vi "Lick.vi"(8 "error in (no error)":errorcluster, 10 "% decrease Thr":dbl[](array[numeric])=[10.0, 10.0, 10.0, 10.0, 10.0], 11 "Licker in":refnum<class "Licker.lvclass">) -> (0 "error out":errorcluster, 1 "Lick?":bool[](array[boolean]), 2 "data":waveform(dbl)[](array[waveform]), 3 "Licker out":refnum<class "Licker.lvclass">)   [LabVIEW 2014, in "Licker.lvclass"]
uses:
  Licker.lvclass
  Licker.lvclass/Licker.ctl
  <vilib>/Analysis/5stat.llb/RMS (DBL).vi
  <vilib>/DAQmx/read.llb/DAQmx Read.vi
  <vilib>/DAQmx/read.llb/DAQmx Read (Analog 1D Wfm NChan NSamp).vi
  <vilib>/Analysis/NI_AALPro.lvlib
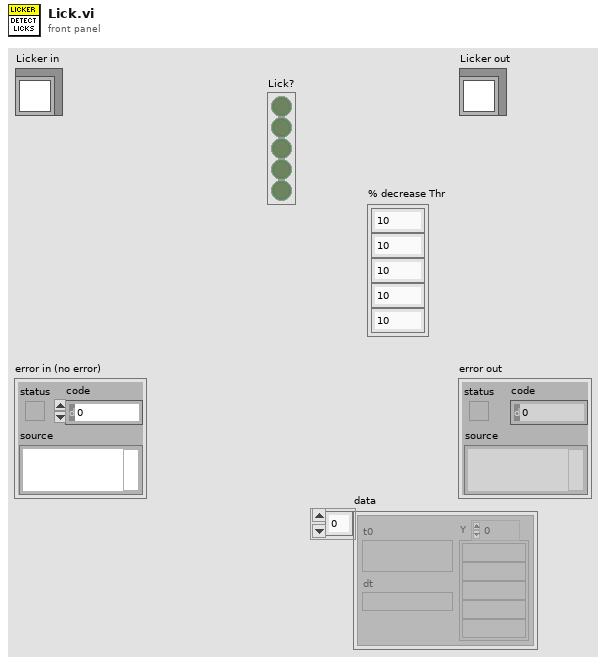
[diagram p1: front panel]
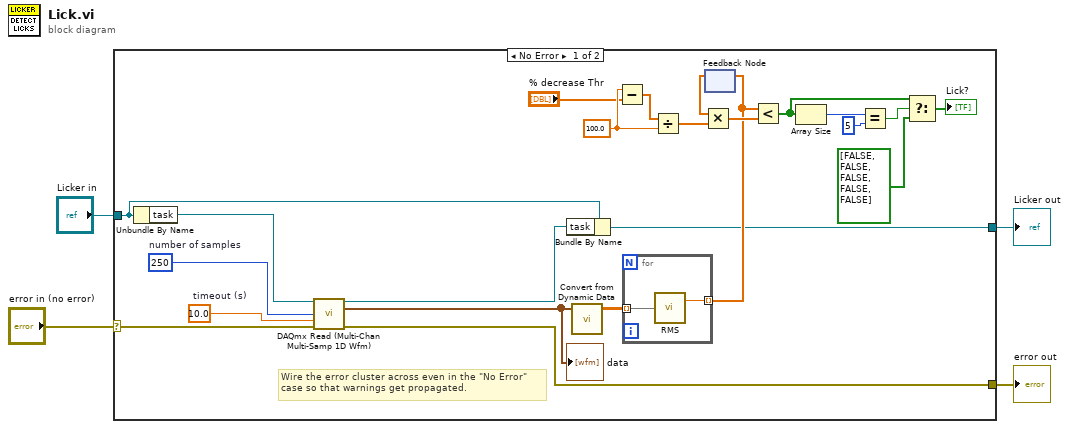
[diagram p0: block diagram]
diagram:
  n1 = case shown="No Error" "error in (no error)" {
    selector: "error in (no error)" -> [w17 w31]
    tunnel: [w16 w31] -> w3
    tunnel: [w13 w30] -> w1
    tunnel: "Licker in" -> [w14 w30]
    frame No Error {
      w18 = 250  # number of samples
      w21 = 100.0 ("y")
      w27 = 10.0  # timeout (s)
      # "Wire the error cluster across even in the \"No Error\"\ncase so that warnings get propagated."
      n2 = Unbundle By Name(w14) -> ("task"=w15:refnum<k21>)
      n3 = call-poly "DAQmx Read (Multi-Chan Multi-Samp 1D Wfm).vi"("task/channels in"=w15, "number of samples per channel"=w18, "timeout"=w27, "error in"=w17) -> ("task out"=w12:refnum<k21>, "data"=w26:waveform(dbl)[], "error out"=w16:errorcluster)  [unwired: 9 in]
      "data" <- w26
      n4 = Bundle By Name(cluster=w14, "task"=w12) -> (w13:refnum<class "Licker.lvclass">)
      n5 = call "Convert from Dynamic Data"("Dynamic Data Type"=w26) -> ("Array"=w25:dbl[][])  [unwired: 3 in]
      n6 = Subtract(x=w21, y="% decrease Thr") -> (x-y=w20:dbl[])
      n7 = for {
        tunnel: w25 -> [w29] mode=indexing
        tunnel: [w28] -> w19 mode=indexing
        n8 = call-poly <vilib>:"RMS.vi"("X"=w29) -> ("rms value"=w28:dbl)  [unwired: 1 out]
      }
      n9 = Divide(x=w20, y=w21) -> (x/y=w22:dbl[])
      n10 = feedback #1() -> (w24:dbl[])  [unwired: 1 in]
      n11 = Multiply(x=w24, y=w22) -> (x*y=w23:dbl[])
      n12 = feedback-in #1(w19) -> ()
      n13 = Less?(x=w19, y=w23) -> (x < y?=w8:bool[])
      n14 = Array Size(array=w8) -> (size(s)=w7:i32)
      n15 = Equal?(x=w7, y=5) -> (x = y?=w5:bool)
      n16 = Select(t=w8, s=w5, f=bool[] [FALSE, FALSE, FALSE, FALSE, FALSE]) -> (s? t:f=→"Lick?":bool[])
    }
    frame Error {
    }
  }
  "error out" <- w3
  "Licker out" <- w1
